vi "worker.vi"(8 "error in (no error)":errorcluster, 9 "Quit":refnum<user-event>, 10 "Message":refnum<user-event>) -> (0 "error out":errorcluster)   [LabVIEW 2015, in "MQTT1.lvclass"]
uses:
  MQTT1.lvclass
  Libraries/mqtt Folder/src/class/mqtt/mqttTXqueue/mqttTXdataQueueFunction.ctl
  Libraries/mqtt Folder/src/class/mqtt/mqttConfigFunction.ctl
  Libraries/mqtt Folder/src/class/mqtt/mqttTXqueue/mqttRXsubscriptionEventFunction.ctl
  Libraries/mqtt Folder/src/class/mqtt/mqtt.lvclass
panel:
  out "RX Topic":string
  out "RX Value":string
  out "messageID":u16
  out "Numeric":i32
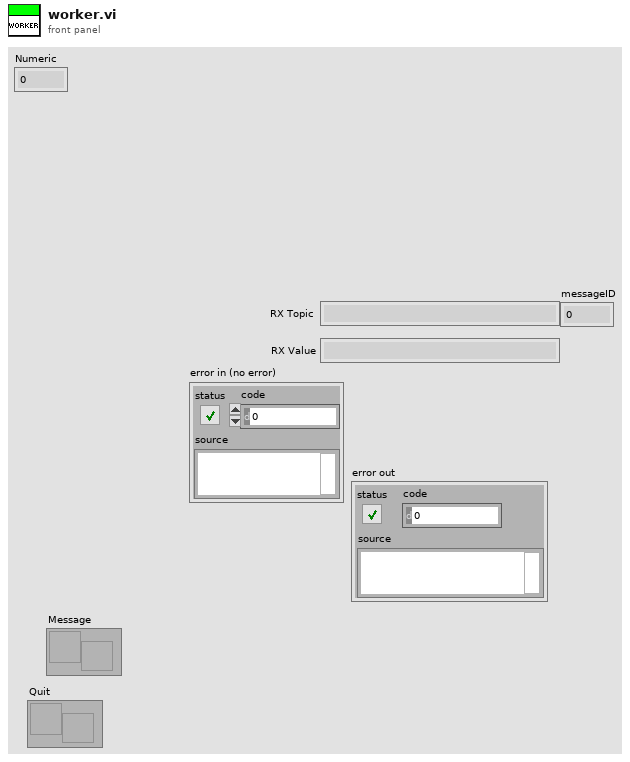
[diagram p1: front panel]
types:
  T1 = typedef "mqttRXsubscriptionEventFunction.ctl" = enum16{"init", "deinit", "getEventRef", "event"}
  T2 = typedef "mqtt.lvclass/mqttConfigFunction.ctl" = enum16{"init", "deinit", "set", "get"}
  T3 = typedef "mqttTXdataQueueFunction.ctl" = enum16{"init", "deinit", "getQueue", "enqueue"}
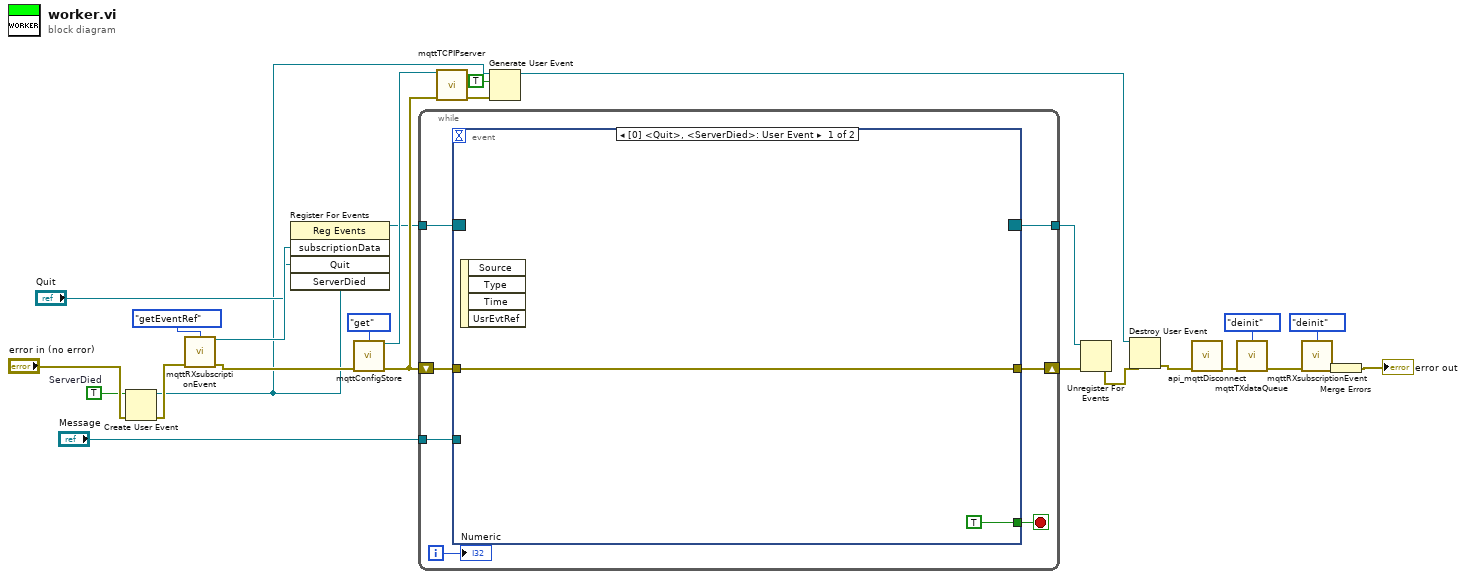
[diagram p0: block diagram]
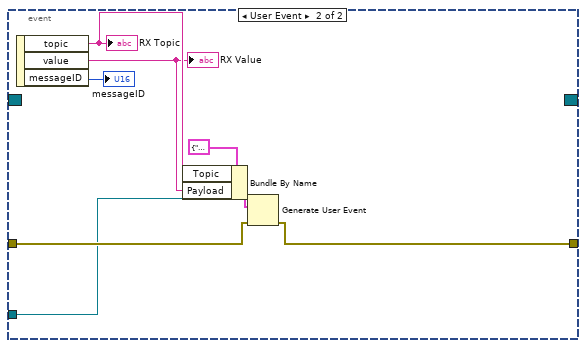
[diagram p2: hidden frame]
diagram:
  w7 = TRUE  # ServerDied
  n1 = Create User Event(user event datatype=w7, error in="error in (no error)") -> (user event=w5:refnum<user-event>, error out=w8:errorcluster)
  n2 = call "mqttRXsubscriptionEvent.vi"("function"=mqttRXsubscriptionEventFunction."getEventRef", "error in (no error)"=w8) -> ("subscriptionData"=w14:refnum<user-event>, "error out"=w13:errorcluster)  [unwired: 12 in]
  n3 = register-events(w14, "Quit", w5) -> (reference out=w21:refnum<event-registration>)  [unwired: 2 in, 1 out]
  n4 = call "mqttConfigStore.vi"("function"=mqttConfigFunction."get", "error in (no error)"=w13) -> ("mqtt.lvclass out"=w24:refnum<class "mqtt.lvclass">, "error out"=w23:errorcluster)  [unwired: 12 in]
  n5 = while {
    shift-right: [w33] -> w17
    shift-left: w23 -> [w32]
    tunnel: w21 -> [w30]
    tunnel: [w28] -> w16
    tunnel: "Message" -> [w27]
    i -> [w29]
    stop <- w31 stop-if-true
    n6 = event shown="[0] <Quit>, <ServerDied>: User Event" {
      selector: w30 -> [_ _]
      dyn-events: [_ _] -> w28
      timeout: _ -> [_ _]
      tunnel: [w34 w41] -> w33
      tunnel: w32 -> [w34 w42]
      tunnel: [TRUE _] -> w31
      tunnel: w27 -> [_ w40]
      event User Event {
        n7 = event-data() -> ()  [unwired: 1 in, 4 out]
      }
      event User Event {
        n8 = event-data() -> ("topic"=w37:string, "value"=w36:string, "messageID"=→"messageID":u16)  [unwired: 1 in]
        "RX Topic" <- w37
        "RX Value" <- w36
        n9 = Bundle By Name(cluster=cluster{"Topic":string, "Payload":string} {"Topic"="", "Payload"=""} ("event data"), "Topic"=w37, "Payload"=w36) -> (w38:cluster{"Topic":string, "Payload":string})
        n10 = Generate User Event(user event=w40, event data cluster=w38, error in=w42) -> (error out=w41:errorcluster)  [unwired: 1 in, 1 out]
      }
    }
    "Numeric" <- w29
  }
  n11 = call "mqttTCPIPserver.vi"("mqtt.lvclass"=w24, "error in (no error)"=w23) -> ("error out"=w6:errorcluster)  [unwired: 12 in, 1 out]
  n12 = Generate User Event(user event=w5, event data cluster=TRUE ("event data"), error in=w6) -> (user event out=w2:refnum<user-event>)  [unwired: 1 in, 1 out]
  n13 = Unregister For Events(event registration refnum=w16, error in=w17) -> (error out=w3:errorcluster)
  n14 = Destroy User Event(user event=w2, error in=w3) -> (error out=w1:errorcluster)
  n15 = call "api_mqttDisconnect.vi"("error in (no error)"=w1) -> ("error out"=w22:errorcluster)  [unwired: 13 in, 1 out]
  n16 = call "mqttTXdataQueue.vi"("function"=mqttTXdataQueueFunction."deinit", "error in (no error)"=w22) -> ("error out"=w19:errorcluster)  [unwired: 12 in, 1 out]
  n17 = call "mqttRXsubscriptionEvent.vi"("function"=mqttRXsubscriptionEventFunction."deinit", "error in (no error)"=w19) -> ("error out"=w18:errorcluster)  [unwired: 12 in, 1 out]
  n18 = Merge Errors(w18) -> (→"error out":errorcluster)
